vi "Initialize Device Core.vi"(8 "error in (no error)":errorcluster, 9 "Reset (F)":bool, 10 "Resource Name":string, 11 "KIT-QVA in":refnum<class "KIT-QVA.lvclass">) -> (0 "error out":errorcluster, 3 "KIT-QVA out":refnum<class "KIT-QVA.lvclass">)   [LabVIEW 2014, in "KIT-QVA.lvlib" / "KIT-QVA.lvclass"]
doc: "Initialize device driver."
uses:
  KIT-QVA.lvclass
  CSPP_Core/Actors/CS++BaseActor/CS++BaseActor.lvclass/CS++BaseActor.ctl
  CSPP_Core/Libraries/Base/Severity.ctl
  KIT-QVA.lvclass/KIT-QVA.ctl
  CSPP_Core/Actors/CS++DeviceActor/CS++DeviceActor.lvclass
  instr.lib/KIT-QV/KIT QV.lvlib
  CSPP_Core/Libraries/Utilities/CS++Utilities.lvlib
  CSPP_Core/Actors/CS++BaseActor/CS++BaseActor.lvclass
  CSPP_Core/Libraries/Base/CS++Base.lvlib
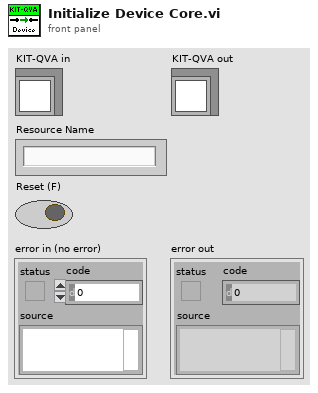
[diagram p1: front panel]
types:
  T1 = typedef "CS++Base.lvlib/Severity.ctl" = enum16{"emergency", "alert", "critical", "error", "warning", "notice", "info", "debug"}
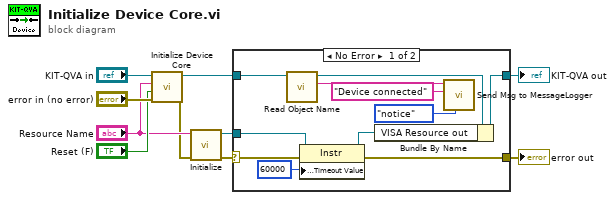
[diagram p0: block diagram]
diagram:
  n1 = call-parent "Initialize Device Core.vi"("error in (no error)"="error in (no error)", "Reset (F)"="Reset (F)", "Resource Name"="Resource Name", "CS++DeviceActor in"="KIT-QVA in") -> ("error out"=w5:errorcluster, "CS++DeviceActor out"=w1:refnum<class "KIT-QVA.lvclass">)  [unwired: 6 in]
  n2 = call "Initialize.vi"("Error In"=w5, "VISA Resource Name"="Resource Name") -> ("Error Out"=w3:errorcluster, "VISA Resource out"=w4:refnum<visa-resource-name>)  [unwired: 8 in]
  n3 = case shown="No Error" w3 {
    selector: w3 -> [w17 w22]
    tunnel: [w21 w23] -> w6
    tunnel: w4 -> [w19 _]
    tunnel: [w16 w22] -> w2
    tunnel: w1 -> [w12 w23]
    frame No Error {
      n4 = call "Read Object Name.vi"("CS++BaseActor in"=w12) -> ("Object Name"=w15:string, "CS++BaseActor out"=w11:refnum<class "KIT-QVA.lvclass">)  [unwired: 8 in, 1 out]
      n5 = property class="Instr"(reference=w19, error in=w17, "General Settings:Timeout Value"=u32 60000) -> (reference out=w18:refnum<visa-resource-name>, error out=w16:errorcluster)
      n6 = Bundle By Name(cluster=w11, "VISA Resource out"=w18) -> (w21:refnum<class "KIT-QVA.lvclass">)
      n7 = call "Send Msg to MessageLogger.vi"("Severity Code (info)"=Severity."notice", "Message Content"="Device connected", "Message Tag"=w15) -> ()  [unwired: 8 in, 1 out]
    }
    frame Error {
    }
  }
  "error out" <- w2
  "KIT-QVA out" <- w6
